vi "Supervisor Log.vi"(9 "Stop Chat":bool, 10 "Send":bool, 11 "Enter Text":string) -> (3 "?":string)   [LabVIEW 2017]
uses:
  <vilib>/OPCUA/controls/Write Status.ctl
  <vilib>/OPCUA/controls/NodeId.ctl
  <vilib>/OPCUA/client/Multiple Write String.vi
  <vilib>/OPCUA/NI OPC UA Client.lvlib
panel:
  out "Log Loop":i32
  out "Send Loop":i32
  in  "Node Status":T1 items=["Good"=0, "Uncertain_InitialValue"=1083310080, "Uncertain_LastUsableValue"=1083179008, "Uncertain_SensorNotAccurate"=1083375616, "Uncertain_EngineeringUnitsExceeded"=1083441152, "Bad_NoCommunication"=2150694912, "Bad_NotReadable"=2151284736, "Bad_NotWritable"=2151350272, "Bad_OutOfRange"=2151415808, "Bad_WaitingForInitialData"=2150760448]
  in  "Time Stamp":timestamp
  in  "Node Status":T1 items=["Good"=0, "Uncertain_InitialValue"=1083310080, "Uncertain_LastUsableValue"=1083179008, "Uncertain_SensorNotAccurate"=1083375616, "Uncertain_EngineeringUnitsExceeded"=1083441152, "Bad_NoCommunication"=2150694912, "Bad_NotReadable"=2151284736, "Bad_NotWritable"=2151350272, "Bad_OutOfRange"=2151415808, "Bad_WaitingForInitialData"=2150760448]
  in  "Time Stamp":timestamp
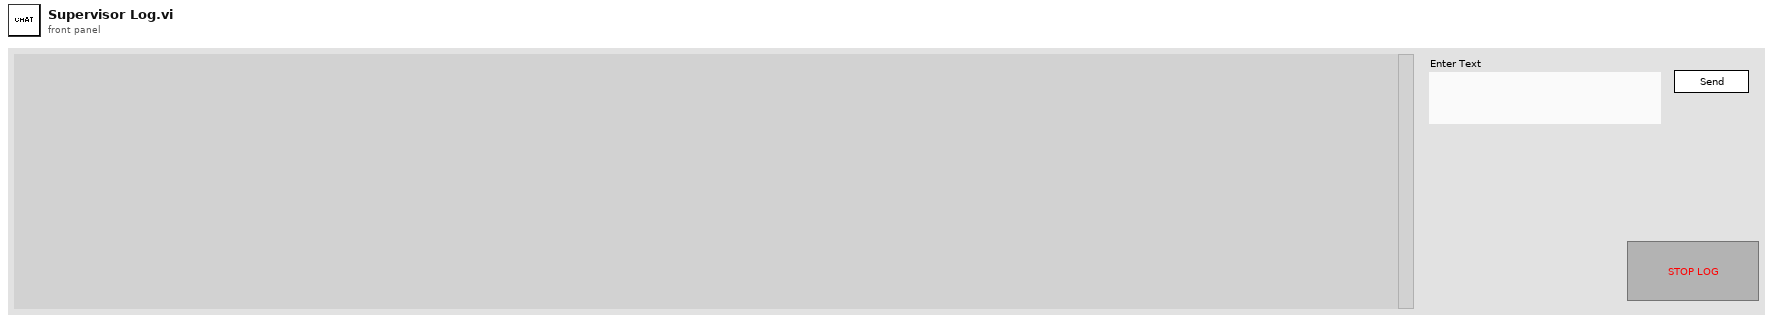
[diagram p1: front panel]
types:
  T1 = typedef "Write Status.ctl" = u32
  T2 = enum16{"open", "replace", "create", "open or create", "replace or create", "replace or create with confirmation"}
  T3 = typedef "OPC UA Client Refnum.ctl" = refnum<k21>
  T4 = typedef "NodeId.ctl" = string
  T5 = cluster{"node ID":T4, "value":string, "timestamp (current time)":timestamp, "node status":T1}
  T6 = cluster{"node ID":T4, "value":string, "timestamp (current time)":timestamp, "node status":T1}[]
  T7 = typedef "Subscription ID.ctl" = u32
  T8 = typedef "Subscription Data Change.ctl" = cluster{"node ID":T4, " value":variant, "timestamp":timestamp, "data type":T9, "status code":T10}
  T9 = typedef "Data Type.ctl" = u16
  T10 = typedef "OPC UA StatusCode.ctl" = u32
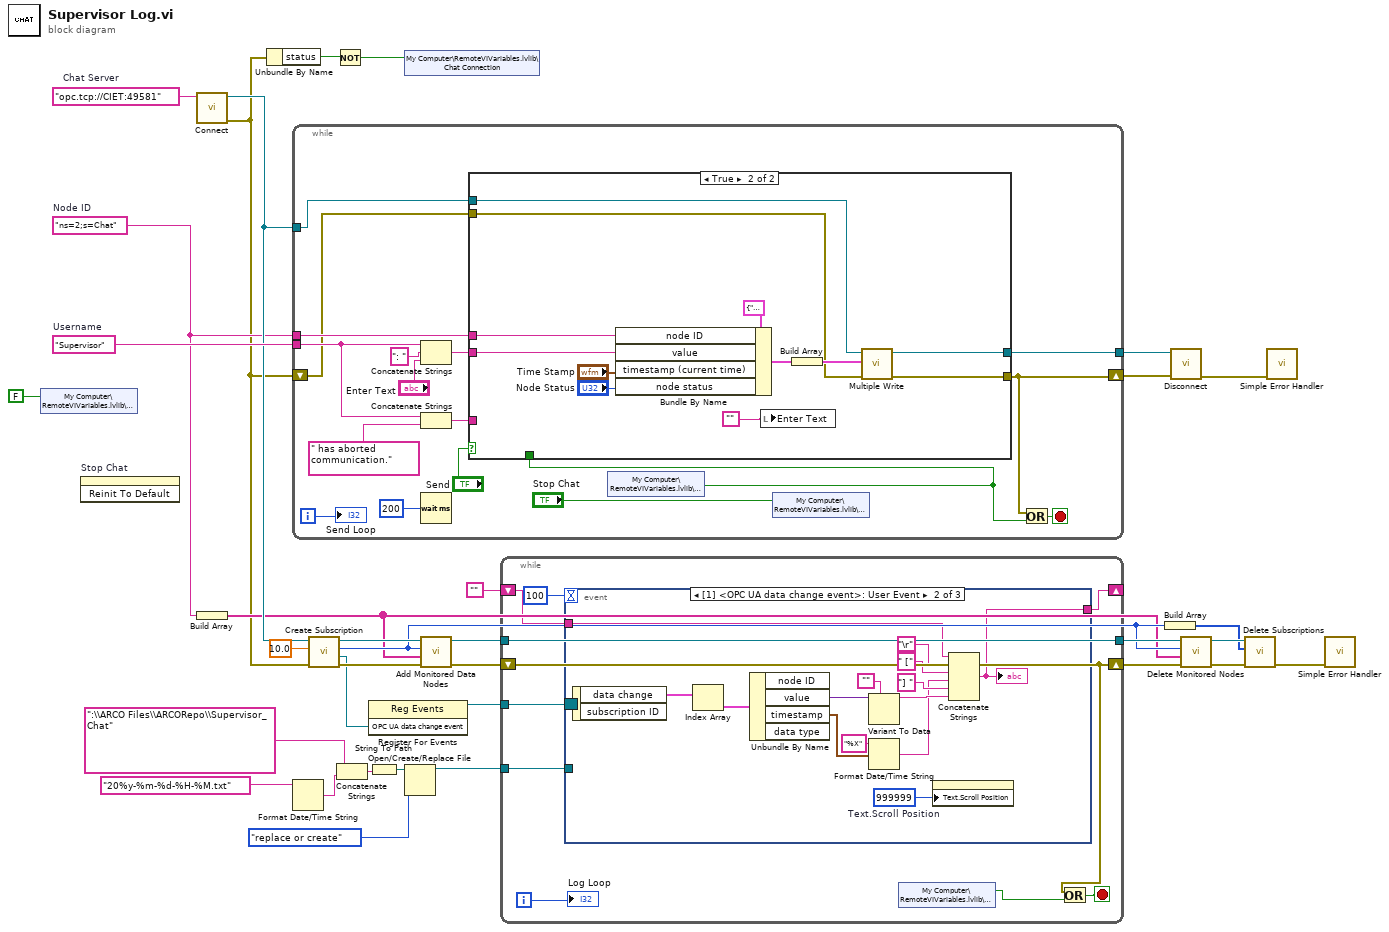
[diagram p0: block diagram]
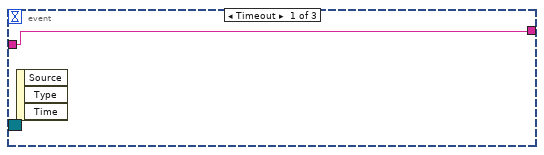
[diagram p2: hidden frame]
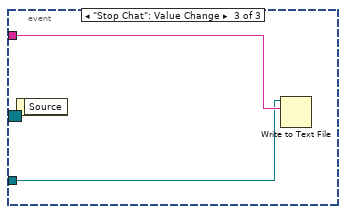
[diagram p3: hidden frame]
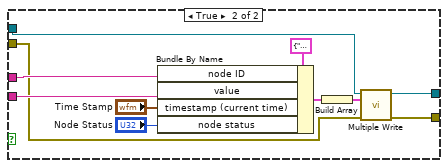
[diagram p5: hidden frame]
diagram:
  w16 = "ns=2;s=Chat"  # Node ID
  w32 = "Supervisor"  # Username
  w33 = "opc.tcp://CIET:49581"  # Chat Server
  n1 = shared-variable "My Computer\\RemoteVIVariables.lvlib\\Stop Chat"(FALSE ("Stop Chat")) -> ()  [unwired: 1 in, 1 out]
  n2 = invoke on="Stop Chat" class="Bool (strict)" method="Reinit To Default"() -> ()  [unwired: 3 in, 3 out]
  n3 = call <vilib>:"Connect.vi"("server endpoint URL"=w33) -> ("error out"=w4:errorcluster, "OPC UA client refnum out"=w31:T3)  [unwired: 8 in, 1 out]
  n4 = Build Array(w16) -> (w15:string[])
  n5 = Unbundle By Name(w4) -> ("status"=w6:bool)
  n6 = while {
    tunnel: w16 -> [w43]
    tunnel: w32 -> [w48]
    tunnel: w31 -> [w41]
    tunnel: [w42] -> w13
    shift-right: [w37] -> w3
    shift-left: w4 -> [w40]
    i -> [w46]
    stop <- w38 stop-if-true
    n7 = Concatenate Strings(w48, ": ", "Enter Text") -> (w44:string)
    n8 = Concatenate Strings(w48, " has aborted communication.") -> (w39:string)
    n9 = Wait (ms)(milliseconds to wait=u32 200) -> ()  [unwired: 1 out]
    n10 = shared-variable "My Computer\\RemoteVIVariables.lvlib\\Stop Chat"() -> (w35:bool)  [unwired: 1 in, 1 out]
    n11 = case shown="True" "Send" {
      tunnel: w44 -> [_ w78]
      tunnel: w43 -> [w56 w77]
      tunnel: [w52 w75] -> w42
      tunnel: [w53 w74] -> w37
      tunnel: w41 -> [w54 w73]
      tunnel: w40 -> [w55 w72]
      tunnel: w35 -> [w58 _]
      tunnel: w39 -> [w57 _]
      frame False {
        n12 = case shown="False" w58 {
          tunnel: w57 -> [_ w66]
          tunnel: w56 -> [_ w65]
          tunnel: w55 -> [w59 w64]
          tunnel: w54 -> [w60 w63]
          tunnel: [w60 w62] -> w52
          tunnel: [w59 w61] -> w53
          frame False {
          }
          frame True {
            n13 = Bundle By Name(cluster=T5 {"node ID"="", "value"="", "timestamp (current time)"=timestamp(0 s since 1904-01-01), "node status"=0} ("request"), "node ID"=w65, "value"=w66, "timestamp (current time)"="Time Stamp", "node status"="Node Status") -> (w69:T5)
            n14 = Build Array(w69) -> (w68:T6)
            n15 = call-poly <vilib>:"Multiple Write.vi"("error in (no error)"=w64, "requests"=w68, "OPC UA client refnum in"=w63) -> ("error out"=w61:errorcluster, "OPC UA client refnum out"=w62:T3)  [unwired: 5 in, 2 out]
          }
        }
      }
      frame True {
        n16 = Bundle By Name(cluster=T5 {"node ID"="", "value"="", "timestamp (current time)"=timestamp(0 s since 1904-01-01), "node status"=0} ("request"), "node ID"=w77, "value"=w78, "timestamp (current time)"="Time Stamp", "node status"="Node Status") -> (w81:T5)
        n17 = local write "Enter Text"("") -> ()
        n18 = Build Array(w81) -> (w80:T6)
        n19 = call-poly <vilib>:"Multiple Write.vi"("error in (no error)"=w72, "requests"=w80, "OPC UA client refnum in"=w73) -> ("error out"=w74:errorcluster, "OPC UA client refnum out"=w75:T3)  [unwired: 5 in, 2 out]
      }
    }
    n20 = shared-variable "My Computer\\RemoteVIVariables.lvlib\\Stop Chat"("Stop Chat") -> ()  [unwired: 1 in, 1 out]
    n21 = Or(x=w37, y=w35) -> (x .or. y?=w38:bool)
    "Send Loop" <- w46
  }
  n22 = Format Date/Time String(time format string (%c)="20%y-%m-%d-%H-%M.txt") -> (date/time string=w10:string)  [unwired: 2 in]
  n23 = call <vilib>:"Create Subscription.vi"("error in (no error)"=w4, "publishing interval (1000 ms)"=10.0, "OPC UA client refnum in"=w31) -> ("error out"=w29:errorcluster, "OPC UA data change event"=w28:refnum<user-event>, "subscription ID out"=w20:T7, "OPC UA client refnum out"=w30:T3)  [unwired: 4 in, 1 out]
  n24 = Not(x=w6) -> (.not. x?=w5:bool)
  n25 = Concatenate Strings(":\\ARCO Files\\ARCORepo\\Supervisor_Chat", w10) -> (w8:string)
  n26 = register-events(w28) -> (reference out=w27:refnum<event-registration>)  [unwired: 2 in, 1 out]
  n27 = String To Path(string=w8) -> (path=w7:path)
  n28 = shared-variable "My Computer\\RemoteVIVariables.lvlib\\Chat Connection"(w5) -> ()  [unwired: 1 in, 1 out]
  n29 = Open/Create/Replace File(file path (use dialog)=w7, operation (0:open)=T2."replace or create") -> (refnum out=w17:refnum<file>)  [unwired: 4 in, 2 out]
  n30 = call <vilib>:"Add Monitored Data Nodes.vi"("error in (no error)"=w29, "node IDs"=w15, "subscription ID in"=w20, "OPC UA client refnum in"=w30) -> ("error out"=w23:errorcluster, "OPC UA client refnum out"=w25:T3)  [unwired: 4 in, 2 out]
  n31 = while {
    tunnel: w27 -> [w93]
    shift-right: [w91] -> _
    shift-left: "" -> [w92]
    tunnel: w25 -> [w90]
    tunnel: [w90] -> w24
    tunnel: w17 -> [w89]
    shift-right: [w85] -> w2
    shift-left: w23 -> [w85]
    i -> [w88]
    stop <- w86 stop-if-true
    n32 = event shown="[1] <OPC UA data change event>: User Event" {
      selector: w93 -> [_ _ _]
      dyn-events: _ -> [_ _ _]
      timeout: 100 -> [_ _ _]
      tunnel: w92 -> [w94 w97 w110]
      tunnel: [w94 w96 _] -> w91
      tunnel: w89 -> [_ _ w109]
      event Timeout {
        n33 = event-data() -> ()  [unwired: 1 in, 3 out]
      }
      event User Event {
        w95 = u32 999999  # Text.Scroll Position
        n34 = event-data() -> ("data change"=w108:T8[])  [unwired: 1 in, 1 out]
        n35 = Index Array(array=w108) -> (element=w107:T8)  [unwired: 1 in]
        n36 = Unbundle By Name(w107) -> ("value"=w106:variant, "timestamp"=w104:timestamp)  [unwired: 2 out]
        n37 = Variant To Data(type="", Variant=w106) -> (data=w102:string)  [unwired: 1 in, 1 out]
        n38 = Format Date/Time String(time format string (%c)="%X", seconds (now)=w104) -> (date/time string=w100:string)  [unwired: 1 in]
        n39 = property class="Str"("Text.Scroll Position"=w95) -> ()  [unwired: 2 in, 2 out]
        n40 = Concatenate Strings(w97, "\r", " [", w100, "] ", w102) -> (w96:string)
        "?" <- w96
      }
      event "Stop Chat": Value Change {
        n41 = event-data() -> ()  [unwired: 1 in, 1 out]
        n42 = Write to Text File(file (use dialog)=w109, text=w110) -> ()  [unwired: 2 in, 3 out]
      }
    }
    n43 = shared-variable "My Computer\\RemoteVIVariables.lvlib\\Stop Chat"() -> (w84:bool)  [unwired: 1 in, 1 out]
    n44 = Or(x=w85, y=w84) -> (x .or. y?=w86:bool)
    "Log Loop" <- w88
  }
  n45 = Build Array(w20) -> (w19:T7[])
  n46 = call <vilib>:"Disconnect.vi"("error in (no error)"=w3, "OPC UA client refnum in"=w13) -> ("error out"=w34:errorcluster)  [unwired: 9 in]
  n47 = call <vilib>:"Delete Monitored Nodes.vi"("error in (no error)"=w2, "node IDs"=w15, "subscription ID in"=w20, "OPC UA client refnum in"=w24) -> ("error out"=w21:errorcluster, "OPC UA client refnum out"=w22:T3)  [unwired: 3 in, 3 out]
  n48 = call <vilib>:"Delete Subscriptions.vi"("error in (no error)"=w21, "subscription IDs"=w19, "OPC UA client refnum in"=w22) -> ("error out"=w18:errorcluster)  [unwired: 6 in, 2 out]
  n49 = call <vilib>:"Simple Error Handler.vi"("error in (no error)"=w34) -> ()  [unwired: 4 in, 5 out]
  n50 = call <vilib>:"Simple Error Handler.vi"("error in (no error)"=w18) -> ()  [unwired: 4 in, 5 out]
